vi "Convert LabVIEW Element to CLFN Element.vi"(5 "Converter Owner":refnum<vi>, 10 "Element Source Terminal":refnum<vi>, 11 "Abstract Param Writer In":refnum<class "Abstract Param Writer.lvclass">) -> (2 "Element Sink Terminal":refnum<vi>, 3 "Abstract Param Writer Out":refnum<class "Abstract Param Writer.lvclass">)   [LabVIEW 2013, in "Abstract Param Writer.lvclass"]
doc: "Copyright (c) 2016 Sze Howe Koh\n\nThis Source Code Form is subject to the terms of the Mozilla Public License, v. 2.0. If a copy of the MPL was not distributed with this file, You can obtain one at http://mozilla.org/MPL/2.0/."
uses:
  Abstract Param Writer.lvclass
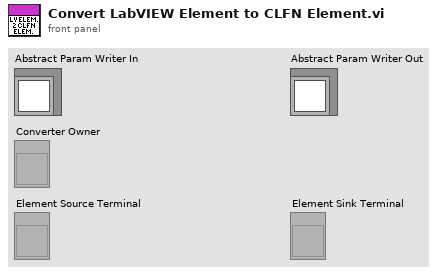
[diagram p1: front panel]
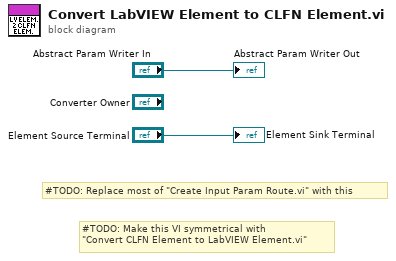
[diagram p0: block diagram]
diagram:
  # "#TODO: Make this VI symmetrical with\n\"Convert CLFN Element to LabVIEW Element.vi\""
  # "#TODO: Replace most of \"Create Input Param Route.vi\" with this"
  "Abstract Param Writer Out" <- "Abstract Param Writer In"
  "Element Sink Terminal" <- "Element Source Terminal"
